vi "Begin.vi"(8 "error in":errorcluster) -> (0 "error out":errorcluster)   [LabVIEW 2015]
doc: "Called before other user functions, this VI is expected to open initial I/O refnums, load in file data, and do all program initialization. Notice that the <B>error out</B> terminal is simply used for data flow. Wiring it to other structures or subVIs ensures that this VI runs first."
uses:
  <vilib>/Rock Robotics/WPI/DriverStation/WPI_DriverStationRobotMode2.ctl
  <vilib>/Rock Robotics/WPI/Joystick/WPI_JoystickDeviceEnum.ctl
  <vilib>/Rock Robotics/WPI/CAN/TalonSRX/WPI_CANTalonSRX_APIFeedbackSelect.ctl
  <vilib>/Rock Robotics/WPI/CAN/TalonSRX/WPI_CANTalonSRX_APIControlMode.ctl
  <vilib>/Rock Robotics/SystemInterfaces/DIO/FPGA_DIOPWMChannel.ctl
  <vilib>/Rock Robotics/WPI/SafetyOutput/WPI_SafetyOutputConfigMenu.ctl
  Robot Global Data.vi
  <vilib>/Rock Robotics/WPI/MotorControl/WPI_MotorControlOpenCANTalonSRX.vi
  <vilib>/Rock Robotics/WPI/MotorControl/WPI_MotorControlOpen VictorSP.vi
  <vilib>/Rock Robotics/WPI/Solenoid/WPI_SolenoidOpenSingle.vi
  <vilib>/Rock Robotics/WPI/RobotDrive/WPI_RobotDriveOpen2MotorWithVictorSP.vi
  <vilib>/Rock Robotics/WPI/Counter/WPI_CounterDigitalInputToDigitalSource.vi
  <vilib>/Rock Robotics/SystemInterfaces/DIO/FPGA_DIOChannel.ctl
  <vilib>/Rock Robotics/WPI/Encoder/WPI_EncoderType.ctl
panel:
  in  "I 4":dbl
  in  "F 4":dbl=0.01
  in  "D 4":dbl caption="D"
  in  "P 4":dbl=1.0 caption="P"
  in  "Reverse Feedback Sensor 4":bool
  in  "I 3":dbl
  in  "F 3":dbl=0.01
  in  "D 3":dbl caption="D"
  in  "P 3":dbl=1.0 caption="P"
  in  "Reverse Feedback Sensor 3":bool
  in  "Encoder Codes Per Rev 3":u16=360
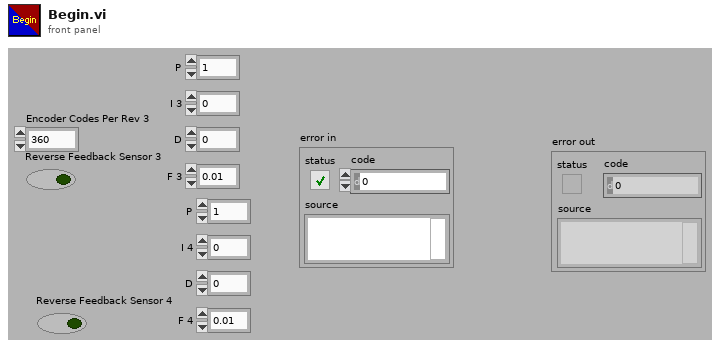
[diagram p1: front panel]
types:
  T1 = typedef "WPI_SafetyOutputConfigMenu.ctl" = enum16{"Enable", "Disable"}
  T2 = typedef "FPGA_DIOPWMChannel.ctl" = enum8{"PWM 0", "PWM 1", "PWM 2", "PWM 3", "PWM 4", "PWM 5", "PWM 6", "PWM 7", "PWM 8", "PWM 9", "PWM MXP 0", "PWM MXP 1", "PWM MXP 2", "PWM MXP 3", "PWM MXP 4", "PWM MXP 5", "PWM MXP 6", "PWM MXP 7", "PWM MXP 8", "PWM MXP 9", "Invalid"}
  T3 = typedef "WPI_CANTalonSRX_APIControlMode.ctl" = enum8{"Percent VBus", "Speed", "Position", "Slave", "Unchanged / Invalid", "Voltage Compensation", "Current", "Motion Profile"}
  T4 = typedef "WPI_CANTalonSRX_APIFeedbackSelect.ctl" = enum16{"Digital Quadrature Encoder", "Analog Potentiometer", "Analog Encoder", "Count on Quad-A (Rising-Edge)", "Count on Quad-A (Falling-Edge)", "CTR Magnetic Enc (Absolute)", "CTR Magnetic Enc (Relative)", "Pulse Width"}
  T5 = typedef "WPI_JoystickDeviceEnum.ctl" = enum16{"USB 0", "USB 1", "USB 2", "USB 3", "USB 4", "USB 5"}
  T6 = typedef "WPI_DriverStationRobotMode2.ctl" = enum16{"Autonomous Disabled", "Autonomous Enabled", "Teleop Disabled", "Teleop Enabled", "Disconnected", "Finish", "Test Disabled", "Test Enabled", "Emergency Stopped"}
  T7 = typedef "WPI_SolenoidDevRef.ctl" = cluster{"DevStatus":errorcluster, "Pneumatics Control Module":u8, "Forward Solenoid Channel":T8, "Reverse Solenoid Channel":T8}
  T8 = typedef "WPI_SolenoidChannel.ctl" = enum8{"Solenoid 0", "Solenoid 1", "Solenoid 2", "Solenoid 3", "Solenoid 4", "Solenoid 5", "Solenoid 6", "Solenoid 7", "Invalid"}
  T9 = typedef "WPI_RobotDriveDevRef.ctl" = cluster{"DevStatus":errorcluster, "Motors[]":T10[], "Square Inputs":bool, "Max Output":dbl}
  T10 = typedef "WPI_MotorControlDeviceRef.ctl" = cluster{"DeviceStatus":errorcluster, "Type":T11, "PWM":cluster{"PWM Channel":T2, "DeadBand":T12}, "CAN":cluster{"Device Number":u8, "Control Mode":T13, "Semaphore":T14, "Max Vout":dbl, "TalonSRX Control Mode":T3}, "Invert":bool}
  T11 = typedef "WPI_MotorControlType.ctl" = enum16{"PWM", "CAN", "CANTalonSRX"}
  T12 = typedef "WPI_PWMDeadband.ctl" = cluster{"Name":string, "maxPositivePwm":i32, "minPositivePwm":i32, "centerPwm":i32, "maxNegativePwm":i32, "minNegativePwm":i32, "angularRange":u16}
  T13 = typedef "WPI_CANJaguar_ControlMode.ctl" = enum8{"Percent VBus", "Current", "Speed", "Position", "Voltage"}
  T14 = typedef "Semaphore RefNum" = refnum<k1>
  T15 = typedef "WPI_JoystickDevRef.ctl" = cluster{"Device":T5}
  T16 = typedef "WPI_EncoderType.ctl" = enum16{"1x", "2x", "4x"}
  T17 = typedef "FPGA_DIOChannel.ctl" = enum8{"DIO 0", "DIO 1", "DIO 2", "DIO 3", "DIO 4", "DIO 5", "DIO 6", "DIO 7", "DIO 8", "DIO 9", "DIO MXP 0", "DIO MXP 1", "DIO MXP 2", "DIO MXP 3", "DIO MXP 4", "DIO MXP 5", "DIO MXP 6", "DIO MXP 7", "DIO MXP 8", "DIO MXP 9", "DIO MXP 10", "DIO MXP 11", "DIO MXP 12", "DIO MXP 13", "DIO MXP 14", "DIO MXP 15", "Invalid"}
  T18 = typedef "WPI_DigitalInputDevRef.ctl" = cluster{"DevStatus":errorcluster, "DIO Channel":T17}
  T19 = typedef "FPGA_CounterEncoderSourceConvertionLVSourceType.ctl" = cluster{"DevStatus":errorcluster, "AnalogTriggerMode?":bool, "DigitalMode":cluster{"DIO Channel":T20}, "AnalogTriggerMode":cluster{"AnalogTriggerIndex":T21, "OutputType":T22}}
  T20 = typedef "FPGA_DIODigitalSourceChannel.ctl" = enum8{"DIO 0", "DIO 1", "DIO 2", "DIO 3", "DIO 4", "DIO 5", "DIO 6", "DIO 7", "DIO 8", "DIO 9", "DIO MXP 0", "DIO MXP 1", "DIO MXP 2", "DIO MXP 3", "DIO MXP 4", "DIO MXP 5", "DIO MXP 6", "DIO MXP 7", "DIO MXP 8", "DIO MXP 9", "DIO MXP 10", "DIO MXP 11", "DIO MXP 12", "DIO MXP 13", "DIO MXP 14", "DIO MXP 15", "Disabled"}
  T21 = typedef "FPGA_AnalogTriggerIndex.ctl" = enum8{"Trig 0", "Trig 1", "Trig 2", "Trig 3", "Trig 4", "Trig 5", "Trig 6", "Trig 7", "Invalid"}
  T22 = typedef "FPGA_AnalogTriggerOutType.ctl" = enum16{"InWindow", "TriggerState", "Rising", "Falling"}
  T23 = typedef "WPI_EncoderDevRef.ctl" = cluster{"DevStatus":errorcluster, "EncoderIndex":T24, "CounterIndex":T25, "DistancePerCount":dbl, "Decoding Type":T16}
  T24 = typedef "FPGA_EncoderIdx.ctl" = enum8{"Enc 0", "Enc 1", "Enc 2", "Enc 3", "Enc 4", "Enc 5", "Enc 6", "Enc 7", "Invalid"}
  T25 = typedef "FPGA_CounterCtrSystemIndex.ctl" = enum8{"Ctr 0", "Ctr 1", "Ctr 2", "Ctr 3", "Ctr 4", "Ctr 5", "Ctr 6", "Ctr 7", "Invalid"}
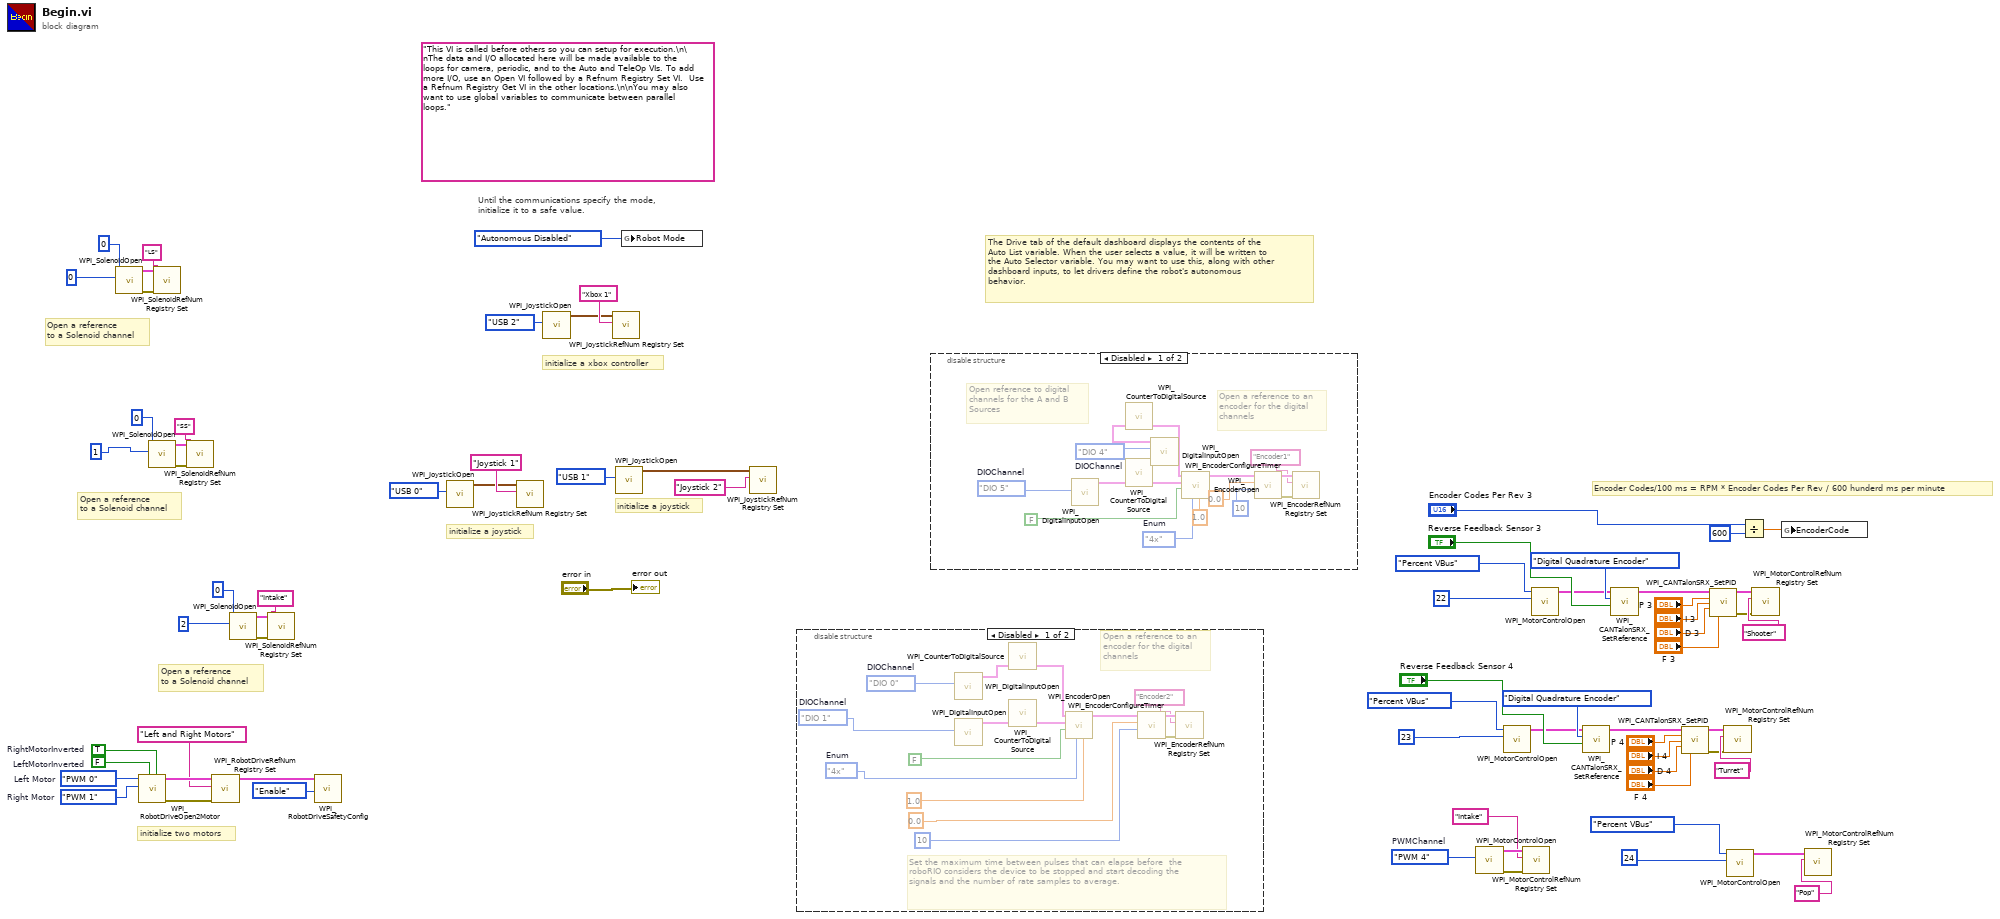
[diagram p0: block diagram]
diagram:
  w3 = FPGA_DIOPWMChannel."PWM 1"  # Right Motor
  w4 = FPGA_DIOPWMChannel."PWM 0"  # Left Motor
  w8 = FALSE  # LeftMotorInverted
  w9 = TRUE  # RightMotorInverted
  w27 = FPGA_DIOPWMChannel."PWM 4"  # PWMChannel
  (unwired) "This VI is called before others so you can setup for execution.\n\nThe data and I/O allocated here will be made available to the loops for camera, periodic, and to the Auto and TeleOp VIs. To add more I/O, use an Open VI followed by a Refnum Registry Set VI.  Use a Refnum Registry Get VI in the other locations.\n\nYou may also want to use global variables to communicate between parallel loops."
  # "initialize two motors"
  # "Open a reference \nto a Solenoid channel"
  # "Open a reference \nto a Solenoid channel"
  # "Open a reference \nto a Solenoid channel"
  # "Encoder Codes/100 ms = RPM * Encoder Codes Per Rev / 600 hunderd ms per minute"
  # "initialize a xbox controller"
  # "The Drive tab of the default dashboard displays the contents of the\nAuto List variable. When the user selects a value, it will be written to\nthe Auto Selector variable. You may want to use this, along with other\ndashboard inputs, to let drivers define the robot's autonomous\nbehavior."
  # "initialize a joystick"
  # "initialize a joystick"
  # "Until the communications specify the mode,\ninitialize it to a safe value."
  n1 = call-poly <vilib>:"WPI_SolenoidOpen.vi"("Solenoid Channel"=0, "Pneumatics Control Module (0)"=0) -> ("error out"=w16:errorcluster, "SolenoidDevRef"=w15:T7)  [unwired: 1 in, 7 out]
  n2 = call-poly <vilib>:"WPI_RobotDriveOpen2Motor.vi"("Right Motor Inverted"=w9, "Left Motor Inverted"=w8, "Right Motor"=w3, "Left Motor"=w4) -> ("error out"=w5:errorcluster, "RobotDriveDevRef"=w7:T9)  [unwired: 1 in, 5 out]
  n3 = call-poly <vilib>:"WPI_SolenoidOpen.vi"("Solenoid Channel"=1, "Pneumatics Control Module (0)"=0) -> ("error out"=w20:errorcluster, "SolenoidDevRef"=w19:T7)  [unwired: 1 in, 7 out]
  n4 = call <vilib>:"WPI_SolenoidRefNum Registry Set.vi"("error in (no error)"=w16, "refnum name"="LS", "SolenoidDevRef"=w15) -> ()  [unwired: 7 in, 2 out]
  n5 = call <vilib>:"WPI_SolenoidRefNum Registry Set.vi"("error in (no error)"=w20, "refnum name"="SS", "SolenoidDevRef"=w19) -> ()  [unwired: 7 in, 2 out]
  n6 = call <vilib>:"WPI_RobotDriveRefNum Registry Set.vi"("error in (no error)"=w5, "refnum name"="Left and Right Motors", "RobotDriveDevRef"=w7) -> ("RobotDriveDevRef"=w2:T9)  [unwired: 1 in, 7 out]
  n7 = call-poly <vilib>:"WPI_SolenoidOpen.vi"("Solenoid Channel"=2, "Pneumatics Control Module (0)"=0) -> ("error out"=w24:errorcluster, "SolenoidDevRef"=w23:T7)  [unwired: 1 in, 7 out]
  n8 = call <vilib>:"WPI_SolenoidRefNum Registry Set.vi"("error in (no error)"=w24, "refnum name"="Intake", "SolenoidDevRef"=w23) -> ()  [unwired: 7 in, 2 out]
  n9 = call <vilib>:"WPI_RobotDriveSafetyConfig.vi"("mode"=WPI_SafetyOutputConfigMenu."Enable", "RobotDriveDevRef"=w2) -> ()  [unwired: 8 in, 2 out]
  n10 = call <vilib>:"WPI_JoystickOpen.vi"("JoystickDevice"=WPI_JoystickDeviceEnum."USB 0") -> ("JoystickDevRef"=w69:T15)  [unwired: 10 in]
  n11 = call <vilib>:"WPI_JoystickRefNum Registry Set.vi"("refnum name"="Joystick 1", "JoystickDevRef"=w69) -> ()  [unwired: 8 in, 2 out]
  n12 = call <vilib>:"WPI_JoystickOpen.vi"("JoystickDevice"=WPI_JoystickDeviceEnum."USB 2") -> ("JoystickDevRef"=w63:T15)  [unwired: 10 in]
  n13 = call <vilib>:"WPI_JoystickRefNum Registry Set.vi"("refnum name"="Xbox 1", "JoystickDevRef"=w63) -> ()  [unwired: 8 in, 2 out]
  n14 = call <vilib>:"WPI_JoystickOpen.vi"("JoystickDevice"=WPI_JoystickDeviceEnum."USB 1") -> ("JoystickDevRef"=w66:T15)  [unwired: 10 in]
  n15 = global write "Robot Global Data.vi" "Robot Mode"(WPI_DriverStationRobotMode2."Autonomous Disabled" ("Robot Mode")) -> ()
  n16 = call <vilib>:"WPI_JoystickRefNum Registry Set.vi"("refnum name"="Joystick 2", "JoystickDevRef"=w66) -> ()  [unwired: 8 in, 2 out]
  n17 = disable-structure shown="Disabled" {
    frame Disabled {
      w76 = WPI_EncoderType."4x"  # Enum
      w78 = FPGA_DIOChannel."DIO 1"  # DIOChannel
      w79 = FPGA_DIOChannel."DIO 0"  # DIOChannel
      # "Set the maximum time between pulses that can elapse before  the roboRIO considers the device to be stopped and start decoding the signals and the number of rate samples to average."
      # "Open a reference to an\nencoder for the digital \nchannels"
      n18 = call <vilib>:"WPI_DigitalInputOpen.vi"("DIO Channel"=w79) -> ("DigitalInputDevRef"=w85:T18)  [unwired: 1 in, 9 out]
      n19 = call <vilib>:"WPI_DigitalInputOpen.vi"("DIO Channel"=w78) -> ("DigitalInputDevRef"=w86:T18)  [unwired: 1 in, 9 out]
      n20 = call-poly <vilib>:"WPI_CounterToDigitalSource.vi"("DigitalInputDevRef"=w85) -> ("Digital Source"=w84:T19)  [unwired: 6 out]
      n21 = call-poly <vilib>:"WPI_CounterToDigitalSource.vi"("DigitalInputDevRef"=w86) -> ("Digital Source"=w87:T19)  [unwired: 6 out]
      n22 = call <vilib>:"WPI_EncoderOpen.vi"("DistancePerCount"=1.0, "Decoding Type"=w76, "Invert Direction (False)"=FALSE, "BSource"=w87, "ASource"=w84) -> ("EncoderDevRef"=w83:T23)  [unwired: 3 in, 3 out]
      n23 = call <vilib>:"WPI_EncoderConfigureTimer.vi"("Number Samples to Average"=10, "Minimum Rate"=0.0, "EncoderDevRef"=w83) -> ("error out"=w82:errorcluster, "EncoderDevRef"=w81:T23)  [unwired: 1 in, 6 out]
      n24 = call <vilib>:"WPI_EncoderRefNum Registry Set.vi"("error in (no error)"=w82, "refnum name"="Encoder2", "EncoderDevRef"=w81) -> ()  [unwired: 7 in, 2 out]
    }
    frame Enabled {
    }
  }
  n25 = disable-structure shown="Disabled" {
    frame Disabled {
      w91 = WPI_EncoderType."4x"  # Enum
      w93 = FPGA_DIOChannel."DIO 5"  # DIOChannel
      w94 = FPGA_DIOChannel."DIO 4"  # DIOChannel
      # "Open a reference to an\nencoder for the digital \nchannels"
      # "Open reference to digital \nchannels for the A and B\nSources"
      n26 = call <vilib>:"WPI_DigitalInputOpen.vi"("DIO Channel"=w93) -> ("DigitalInputDevRef"=w101:T18)  [unwired: 1 in, 9 out]
      n27 = call-poly <vilib>:"WPI_CounterToDigitalSource.vi"("DigitalInputDevRef"=w101) -> ("Digital Source"=w102:T19)  [unwired: 6 out]
      n28 = call <vilib>:"WPI_DigitalInputOpen.vi"("DIO Channel"=w94) -> ("DigitalInputDevRef"=w100:T18)  [unwired: 1 in, 9 out]
      n29 = call-poly <vilib>:"WPI_CounterToDigitalSource.vi"("DigitalInputDevRef"=w100) -> ("Digital Source"=w99:T19)  [unwired: 6 out]
      n30 = call <vilib>:"WPI_EncoderOpen.vi"("DistancePerCount"=1.0, "Decoding Type"=w91, "Invert Direction (False)"=FALSE, "BSource"=w102, "ASource"=w99) -> ("EncoderDevRef"=w98:T23)  [unwired: 3 in, 3 out]
      n31 = call <vilib>:"WPI_EncoderConfigureTimer.vi"("Number Samples to Average"=10, "Minimum Rate"=0.0, "EncoderDevRef"=w98) -> ("error out"=w97:errorcluster, "EncoderDevRef"=w96:T23)  [unwired: 1 in, 6 out]
      n32 = call <vilib>:"WPI_EncoderRefNum Registry Set.vi"("error in (no error)"=w97, "refnum name"="Encoder1", "EncoderDevRef"=w96) -> ()  [unwired: 7 in, 2 out]
    }
    frame Enabled {
    }
  }
  n33 = call-poly <vilib>:"WPI_MotorControlOpen.vi"("PWM Channel"=w27) -> ("error out"=w29:errorcluster, "MotorControlDeviceRef"=w28:T10)  [unwired: 9 in]
  n34 = call-poly <vilib>:"WPI_MotorControlOpen.vi"("Device Number"=23, "Control Mode"=WPI_CANTalonSRX_APIControlMode."Percent VBus") -> ("MotorControlDeviceRef"=w41:T10)  [unwired: 3 in, 6 out]
  n35 = call <vilib>:"WPI_MotorControlRefNum Registry Set.vi"("error in (no error)"=w29, "refnum name"="Intake", "MotorControlDevRef"=w28) -> ()  [unwired: 7 in, 2 out]
  n36 = call-poly <vilib>:"WPI_MotorControlOpen.vi"("Device Number"=22, "Control Mode"=WPI_CANTalonSRX_APIControlMode."Percent VBus") -> ("MotorControlDeviceRef"=w54:T10)  [unwired: 3 in, 6 out]
  n37 = call <vilib>:"WPI_CANTalonSRX_SetReference.vi"("Reverse Feedback Sensor"="Reverse Feedback Sensor 4", "Feedback Reference"=WPI_CANTalonSRX_APIFeedbackSelect."Digital Quadrature Encoder", "CAN Talon SRX Ref"=w41) -> ("CAN Talon SRX Ref"=w40:T10)  [unwired: 7 in, 1 out]
  n38 = call <vilib>:"WPI_CANTalonSRX_SetReference.vi"("Reverse Feedback Sensor"="Reverse Feedback Sensor 3", "Feedback Reference"=WPI_CANTalonSRX_APIFeedbackSelect."Digital Quadrature Encoder", "CAN Talon SRX Ref"=w54) -> ("CAN Talon SRX Ref"=w53:T10)  [unwired: 7 in, 1 out]
  n39 = call <vilib>:"WPI_CANTalonSRX_SetPID.vi"("CAN Talon SRX Ref"=w40, "P"="P 4", "I"="I 4", "D"="D 4", "F"="F 4") -> ("CAN Talon SRX Ref"=w37:T10, "error out"=w35:errorcluster)  [unwired: 9 in]
  n40 = call <vilib>:"WPI_CANTalonSRX_SetPID.vi"("CAN Talon SRX Ref"=w53, "P"="P 3", "I"="I 3", "D"="D 3", "F"="F 3") -> ("CAN Talon SRX Ref"=w49:T10, "error out"=w47:errorcluster)  [unwired: 9 in]
  n41 = call <vilib>:"WPI_MotorControlRefNum Registry Set.vi"("error in (no error)"=w35, "refnum name"="Turret", "MotorControlDevRef"=w37) -> ()  [unwired: 7 in, 2 out]
  n42 = call-poly <vilib>:"WPI_MotorControlOpen.vi"("Device Number"=24, "Control Mode"=WPI_CANTalonSRX_APIControlMode."Percent VBus") -> ("MotorControlDeviceRef"=w25:T10)  [unwired: 3 in, 6 out]
  n43 = Divide(x="Encoder Codes Per Rev 3", y=u16 600) -> (x/y=w50:dbl)
  n44 = call <vilib>:"WPI_MotorControlRefNum Registry Set.vi"("error in (no error)"=w47, "refnum name"="Shooter", "MotorControlDevRef"=w49) -> ()  [unwired: 7 in, 2 out]
  n45 = global write "Robot Global Data.vi" "EncoderCode"(w50) -> ()
  n46 = call <vilib>:"WPI_MotorControlRefNum Registry Set.vi"("refnum name"="Pop", "MotorControlDevRef"=w25) -> ()  [unwired: 8 in, 2 out]
  "error out" <- "error in"
